vi "test-linear-filter-test-03-derivF.vi"(11 "Input":dbl) -> (3 "Output":dbl)   [LabVIEW 2019]
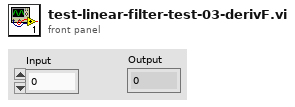
[diagram p1: front panel]
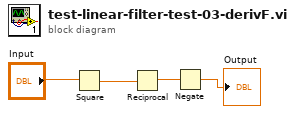
[diagram p0: block diagram]
diagram:
  n1 = Square(x="Input") -> (x^2=w4:dbl)
  n2 = Reciprocal(x=w4) -> (1/x=w1:dbl)
  n3 = Negate(x=w1) -> (-x=→"Output":dbl)
